vi "UDP - Open Connection.vi"(7 "CMD":T1={"UDP CMD"={"IP"="", "CMD"=enum."Stop", "Port"="", "Datalog?"=FALSE, "Float"=0.0}, "Unit?"=FALSE, "Read Unit"=[], "Trig?"=FALSE, "UDP Info"=[], "DataLogger"=[], "VISA Ref"=refnum, "Float"=0.0, "Data"={"Test"={"Target Load"=0.0, "Target Disp"=0.0, "Rate"=0.0, "Speed"=0.0}, "Sensor"={"Name"=[], "Unit"=[], "Decimal Point"=[], "Ch Log"=[], "H Alarm"=[], "L Alarm"=[], "H Limit"=[], "L Limit"=[], "Filter"=[], "Gain"=[], "Calib Type"=[]}, "PID"={"SP"=-2.7823365e-08, "PV"=-3.023652e-13, "kP"=8.5432666e-24, "kI"=2.29252e-41, "kD"=1.570387e-38, "FF"=25.0, "Err Band"=0.0, "Max"=15, "Min"=-7, "Ts"=1886611780, "Out"=0, "Mode"=0}, "ADC"={"Active Ch"=[255, 255, 255, 0, 0, 0, 0, 0], "Filter Type"=2, "Post Filter"=[1, 1, 1, 1, 0, 200, 66, 184], "Gain"=[0, 0, 0, 0, 0, 122, 68, 0], "FS"=32, "IntOC"=0, "IntFC"=255, "SysOC"=255, "Cofficient"=[1.0, 1.0, 1.0, 1.0, 1.0, 1.0, 1.0, 1.0], "K"=[1.2450000047683716, 1.2450000047683716], "Max"=1048576}, "System"={"Out Type"=0, "Inverse"=0, "Monitor"=0, "Reserve"=0, "ACC Time"=0, "Pulse Rev"=0, "Stroke"=0, "Auto Off"=0, "Gear Ratio"=0.0, "Pitch"=0.0, "Max Speed"=0, "Jog Speed"=0, "Disp Coff"=0.0, "Max Load"=0}, "Index"=enum."Ch1", "Datalog"=enum."Empty"}, "UDP Event Ref"=refnum, "UDP ref"=refnum, "Read Sensor"=0}, 8 "error in":errorcluster, 11 "UDP Info":T5={"IP Address"="192.168.88.49", "port"="", "UDP ref"=refnum}) -> (0 "error out":errorcluster, 3 "UDP Info Out":T5, 5 "?":T1={"UDP CMD"={"IP"="", "CMD"=enum."Stop", "Port"="", "Datalog?"=FALSE, "Float"=0.0}, "Unit?"=FALSE, "Read Unit"=[], "Trig?"=FALSE, "UDP Info"=[], "DataLogger"=[], "VISA Ref"=refnum, "Float"=0.0, "Data"={"Test"={"Target Load"=0.0, "Target Disp"=0.0, "Rate"=0.0, "Speed"=0.0}, "Sensor"={"Name"=[], "Unit"=[], "Decimal Point"=[], "Ch Log"=[], "H Alarm"=[], "L Alarm"=[], "H Limit"=[], "L Limit"=[], "Filter"=[], "Gain"=[], "Calib Type"=[]}, "PID"={"SP"=-2.7823365e-08, "PV"=-3.023652e-13, "kP"=8.5432666e-24, "kI"=2.29252e-41, "kD"=1.570387e-38, "FF"=25.0, "Err Band"=0.0, "Max"=15, "Min"=-7, "Ts"=1886611780, "Out"=0, "Mode"=0}, "ADC"={"Active Ch"=[255, 255, 255, 0, 0, 0, 0, 0], "Filter Type"=2, "Post Filter"=[1, 1, 1, 1, 0, 200, 66, 184], "Gain"=[0, 0, 0, 0, 0, 122, 68, 0], "FS"=32, "IntOC"=0, "IntFC"=255, "SysOC"=255, "Cofficient"=[1.0, 1.0, 1.0, 1.0, 1.0, 1.0, 1.0, 1.0], "K"=[1.2450000047683716, 1.2450000047683716], "Max"=1048576}, "System"={"Out Type"=0, "Inverse"=0, "Monitor"=0, "Reserve"=0, "ACC Time"=0, "Pulse Rev"=0, "Stroke"=0, "Auto Off"=0, "Gear Ratio"=0.0, "Pitch"=0.0, "Max Speed"=0, "Jog Speed"=0, "Disp Coff"=0.0, "Max Load"=0}, "Index"=enum."Ch1", "Datalog"=enum."Empty"}, "UDP Event Ref"=refnum, "UDP ref"=refnum, "Read Sensor"=0})   [LabVIEW 2019]
uses:
  Controls/Communications - Data Structure.ctl
  Controls/FTDI - Communication.ctl
  Controls/UDP - Command.ctl
  Controls/Communication - Write Data.ctl
  Controls/UDP - Communication.ctl
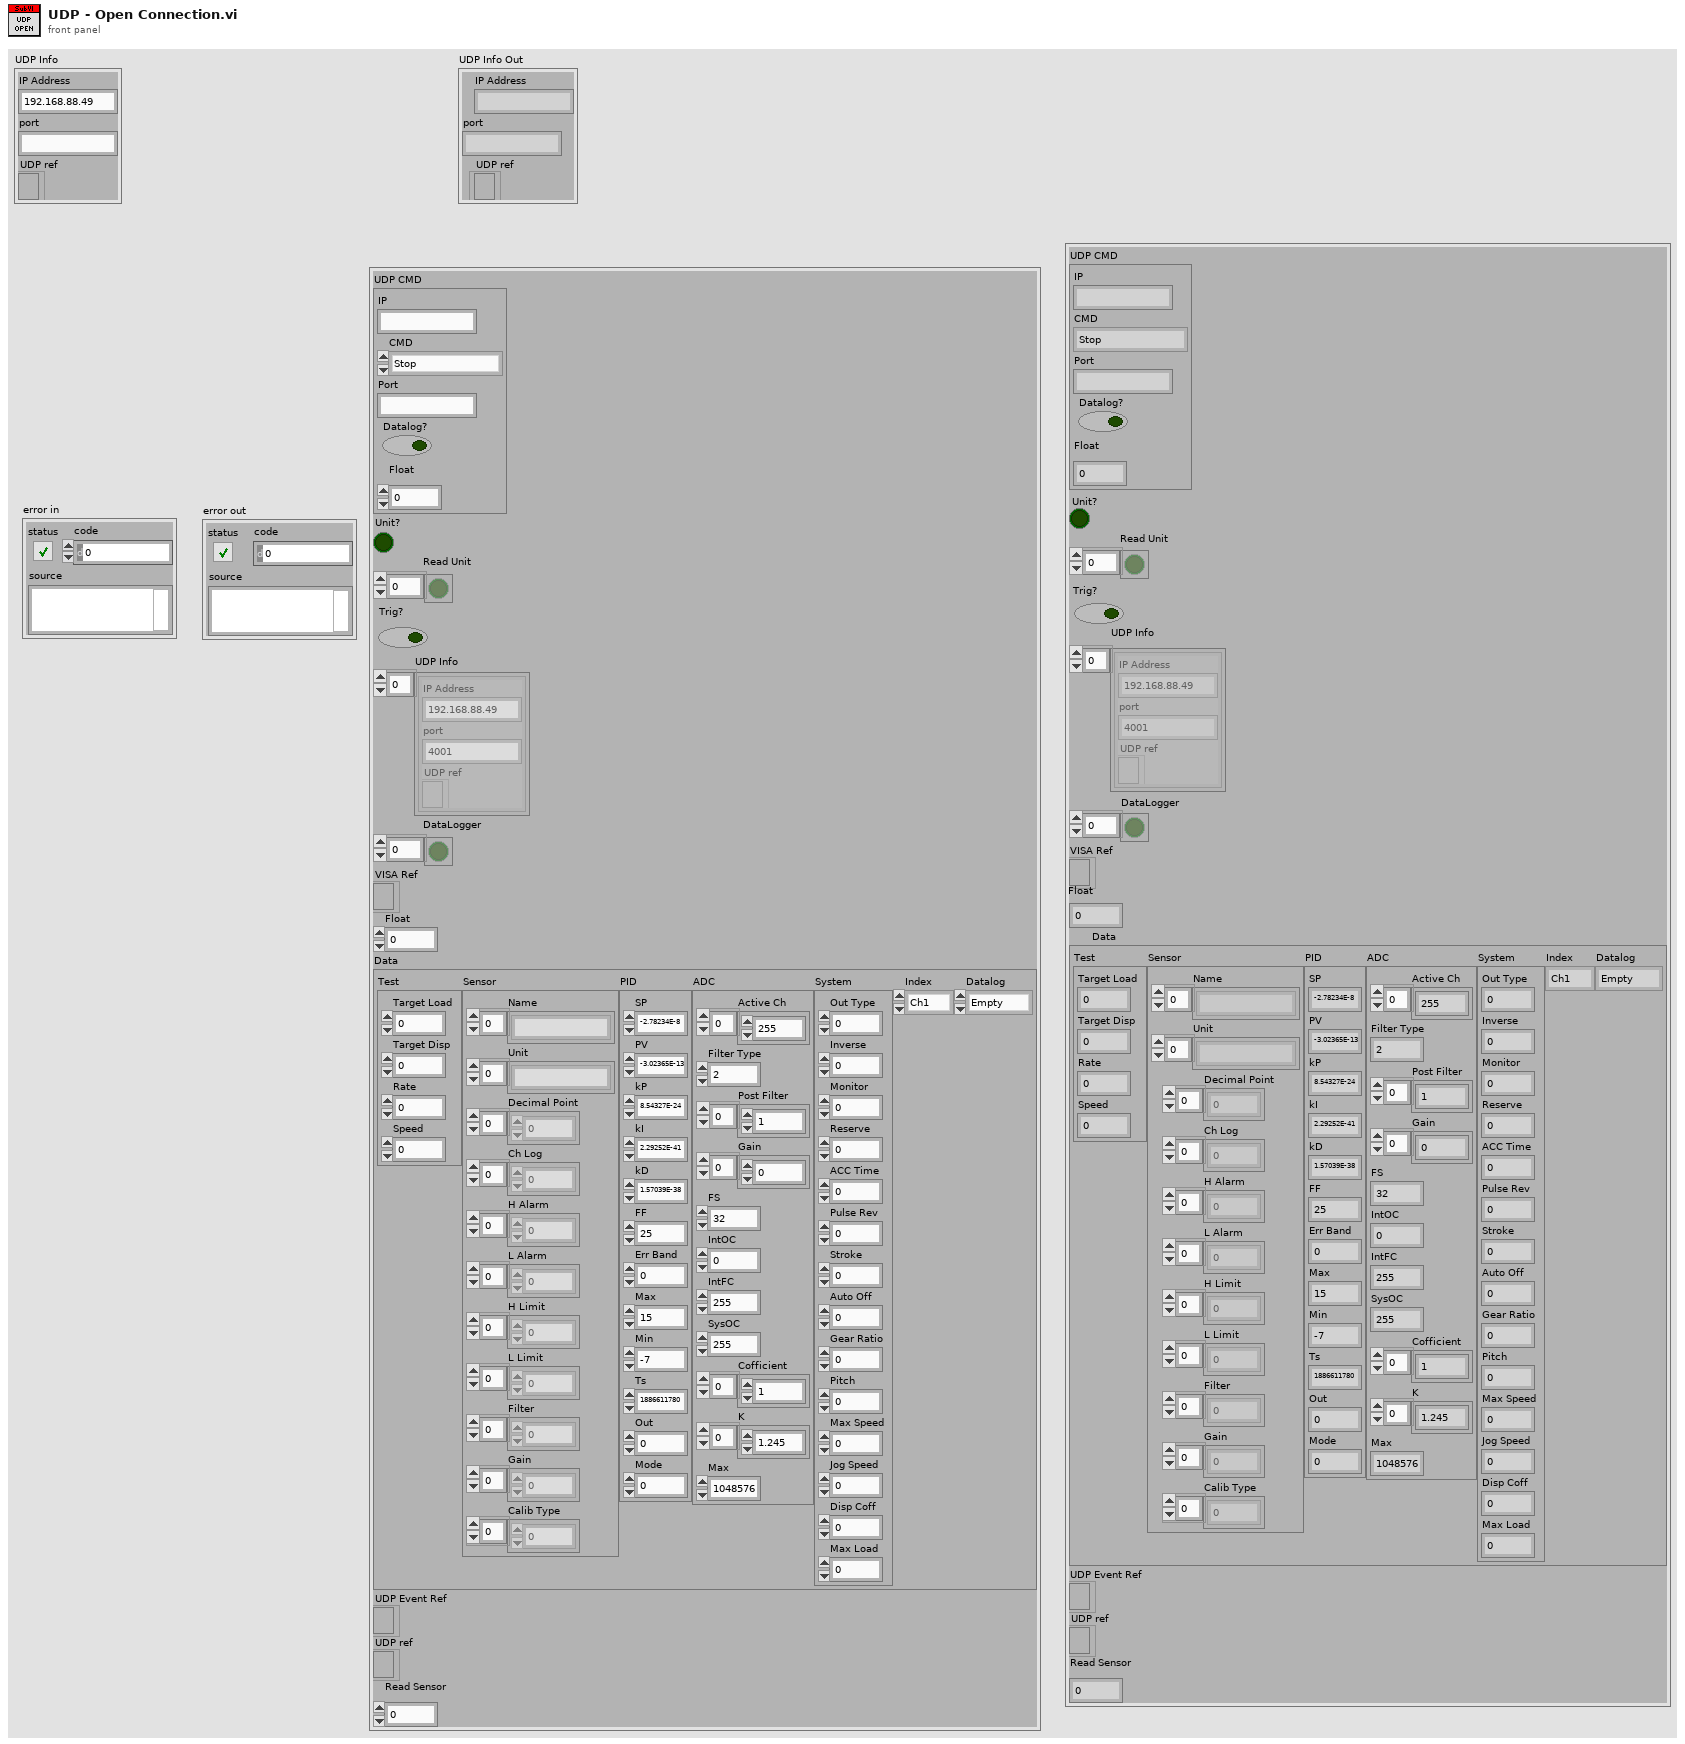
[diagram p1: front panel]
types:
  T1 = typedef "Communications - Data Structure.ctl" = cluster{"UDP CMD":T2, "Unit?":bool, "Read Unit":bool[], "Trig?":bool, "UDP Info":cluster{"IP Address":string, "port":string, "UDP ref":refnum<k16>}[], "DataLogger":bool[], "VISA Ref":refnum<event-registration>, "Float":sgl, "Data":T4, "UDP Event Ref":refnum<event-registration>, "UDP ref":refnum<k16>, "Read Sensor":u8}
  T2 = typedef "FTDI - Communication.ctl" = cluster{"IP":string, "CMD":T3, "Port":string, "Datalog?":bool, "Float":dbl}
  T3 = typedef "UDP - Command.ctl" = enum16{"Stop", "Jog Up", "Jog Down", "Ramp Up", "Ramp Down", "PID Target", "PID Ramp", "Disp Run", "Read Ch Data", "Zero Channel", "Zero Disp", "Read Sensor", "Write Sensor", "Read ADC", "Write ADC", "Read PID", "Write PID", "Read Test", "Write Test", "Read System", "Write System", "Read Datalog", "Read Datalog Sensor"}
  T4 = typedef "Communication - Write Data.ctl" = cluster{"Test":cluster{"Target Load":sgl, "Target Disp":sgl, "Rate":sgl, "Speed":sgl}, "Sensor":cluster{"Name":string[], "Unit":string[], "Decimal Point":u8[], "Ch Log":u8[], "H Alarm":u8[], "L Alarm":u8[], "H Limit":sgl[], "L Limit":sgl[], "Filter":u8[], "Gain":u8[], "Calib Type":u32[]}, "PID":cluster{"SP":sgl, "PV":sgl, "kP":sgl, "kI":sgl, "kD":sgl, "FF":sgl, "Err Band":sgl, "Max":i32, "Min":i32, "Ts":u32, "Out":i32, "Mode":u8}, "ADC":cluster{"Active Ch":u8[], "Filter Type":u8, "Post Filter":u8[], "Gain":u8[], "FS":u16, "IntOC":u8, "IntFC":u8, "SysOC":u8, "Cofficient":dbl[], "K":dbl[], "Max":i32}, "System":cluster{"Out Type":u8, "Inverse":u8, "Monitor":u8, "Reserve":u8, "ACC Time":u32, "Pulse Rev":u32, "Stroke":u32, "Auto Off":u32, "Gear Ratio":sgl, "Pitch":sgl, "Max Speed":u32, "Jog Speed":u32, "Disp Coff":sgl, "Max Load":u32}, "Index":enum16{"Ch1", "Ch2", "Ch3", "Ch4", "Ch5", "Ch6", "Ch7", "Ch8", "Ch9", "Ch10", "Ch11", "Ch12", "Ch13", "Ch14", "Ch15", "Ch16"}, "Datalog":enum16{"Ch1-Ch16", "Ch17-Ch32", "Ch32-Ch48", "Ch49-Ch64", "Empty"}}
  T5 = cluster{"IP Address":string, "port":string, "UDP ref":refnum<k16>}
  T6 = cluster{"IP Address":string, "port":string, "UDP ref":refnum<k16>}[]
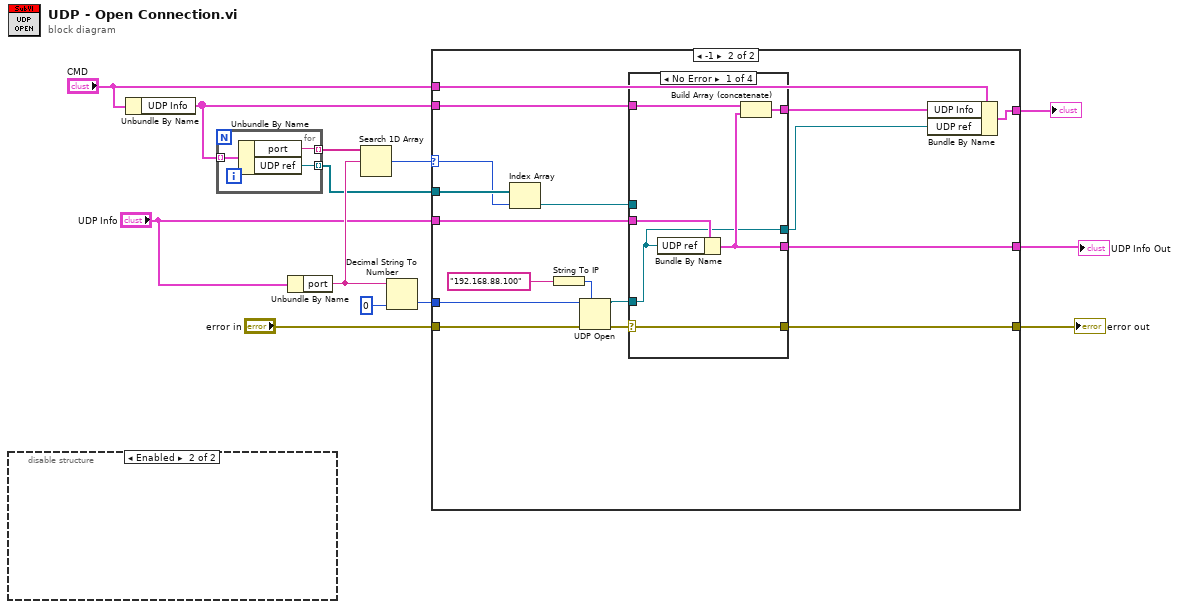
[diagram p0: block diagram]
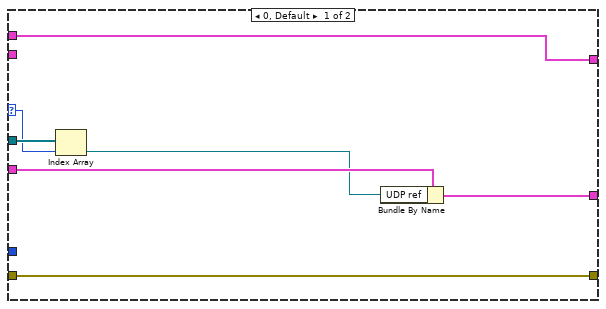
[diagram p2: hidden frame]
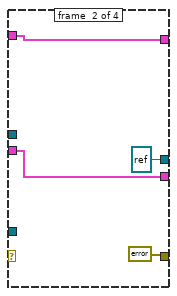
[diagram p3: hidden frame]
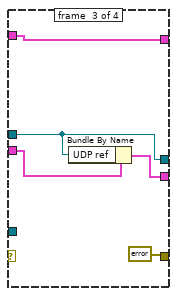
[diagram p4: hidden frame]
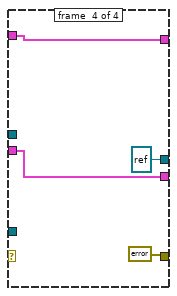
[diagram p5: hidden frame]
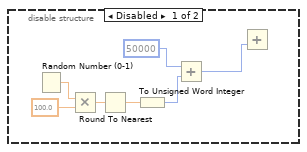
[diagram p6: hidden frame]
diagram:
  n1 = disable-structure shown="Enabled" {
    frame Disabled {
      n2 = Random Number (0-1)() -> (number: 0 to 1=w16:dbl)
      n3 = Multiply(x=w16, y=100.0) -> (x*y=w17:dbl)
      n4 = Round To Nearest(number=w17) -> (nearest integer value=w15:dbl)
      n5 = To Unsigned Word Integer(number=w15) -> (unsigned 16bit integer=w14:u16)
      n6 = Add(x=u16 50000, y=w14) -> (x+y=w19:u16)
      n7 = Add(y=w19) -> ()  [unwired: 1 in, 1 out]
    }
    frame Enabled {
    }
  }
  n8 = Unbundle By Name("CMD") -> ("UDP Info"=w3:T6)
  n9 = for {
    tunnel: w3 -> [w23] mode=indexing
    tunnel: [w22] -> w9 mode=indexing
    tunnel: [w21] -> w6 mode=indexing
    n10 = Unbundle By Name(w23) -> ("port"=w22:string, "UDP ref"=w21:refnum<k16>)
  }
  n11 = Unbundle By Name("UDP Info") -> ("port"=w8:string)
  n12 = Search 1D Array(1D array=w9, element=w8) -> (index of element=w7:i32)  [unwired: 1 in]
  n13 = Decimal String To Number(string=w8, default (0L)=u16 0 ("port")) -> (number=w11:u16)  [unwired: 1 in, 1 out]
  n14 = case shown="-1" w7 {
    selector: w7 -> [w29 w40]
    tunnel: [w28 w47] -> w13
    tunnel: w11 -> [_ w43]
    tunnel: "error in" -> [w28 w42]
    tunnel: w6 -> [w30 w41]
    tunnel: "CMD" -> [w24 w38]
    tunnel: "UDP Info" -> [w27 w35]
    tunnel: [w25 w33] -> w4
    tunnel: w3 -> [_ w36]
    tunnel: [w24 w37] -> w2
    frame 0, Default {
      n15 = Index Array(array=w30, index=w29) -> (element=w26:refnum<k16>)
      n16 = Bundle By Name(cluster=w27, "UDP ref"=w26) -> (w25:T5)
    }
    frame -1 {
      n17 = Index Array(array=w41, index=w40) -> (element=w39:refnum<k16>)
      n18 = String To IP(1:"192.168.88.100" ("name")) -> (0:w44:u32)
      n19 = UDP Open(7:w44, 8:w42, 11:w43) -> (port=w45:refnum<k16>, 0:w46:errorcluster)  [unwired: 2 in, 1 out]
      n20 = case shown="No Error" w46 {
        selector: w46 -> [w53 _ _ _]
        tunnel: w45 -> [w48 _ _ _]
        tunnel: [w53 errorcluster {"status"=FALSE, "code"=0, "source"=""} ("error IO") errorcluster {"status"=FALSE, "code"=0, "source"=""} ("error IO") errorcluster {"status"=FALSE, "code"=0, "source"=""} ("error IO")] -> w47
        tunnel: w39 -> [_ _ w58 _]
        tunnel: w36 -> [w52 w55 w61 w64]
        tunnel: w35 -> [w51 w56 w59 w65]
        tunnel: [w50 w55 w61 w64] -> w34
        tunnel: [w49 w56 w60 w65] -> w33
        tunnel: [w48 refnum<k16> refnum ("port") w58 refnum<k16> refnum ("UDP ref")] -> w32
        frame #0 {
          n21 = Bundle By Name(cluster=w51, "UDP ref"=w48) -> (w49:T5)
          n22 = Build Array (concatenate)(w52, w49) -> (w50:T6)
        }
        frame #1 {
        }
        frame #2 {
          n23 = Bundle By Name(cluster=w59, "UDP ref"=w58) -> (w60:T5)
        }
        frame #3 {
        }
      }
      n24 = Bundle By Name(cluster=w38, "UDP Info"=w34, "UDP ref"=w32) -> (w37:T1)
    }
  }
  "error out" <- w13
  "UDP Info Out" <- w4
  "?" <- w2
